vi "TIO Data Stream Parse timebase Info.vi"(8 "timebases in":T2(array[cluster]), 11 "timebase info raw":string="\u0001\u0000\u0001\u0002 \u0006\u001c\u0006\u0000\u0000\u0000\u0000Ð\u0012\u0013\u0000è\u0003\u0000\u0000\u0001\u0000\u0000\u0000\u0017·Q8\u0001\u0000\u0000\u0000?\u0000\u0016\u0000\u0011P6W462 ") -> (0 "timebases out":T2(array[cluster]))   [LabVIEW 2012]
panel:
  out "timebase info":T1
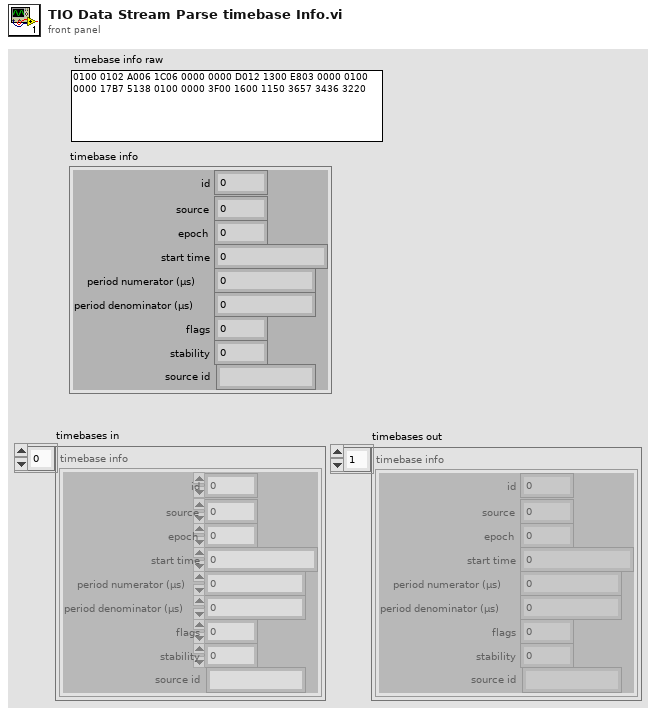
[diagram p1: front panel]
types:
  T1 = cluster{"id":u16, "source":u8, "epoch":u8, "start time":u64, "period numerator (µs)":u32, "period denominator (µs)":u32, "flags":u32, "stability":sgl, "source id":string}
  T2 = cluster{"id":u16, "source":u8, "epoch":u8, "start time":u64, "period numerator (µs)":u32, "period denominator (µs)":u32, "flags":u32, "stability":sgl, "source id":string}[]
  T3 = enum16{"big-endian, network order", "native, host order", "little-endian"}
  T4 = cluster{"u16":u16, "u8":u8, "u8":u8, "u64":u64, "u32":u32, "u32":u32, "u32":u32, "f32":sgl}
  T5 = cluster{"u16":u16, "u8":u8, "u8":u8, "u64":u64, "u32":u32, "u32":u32, "u32":u32, "f32":sgl, string}
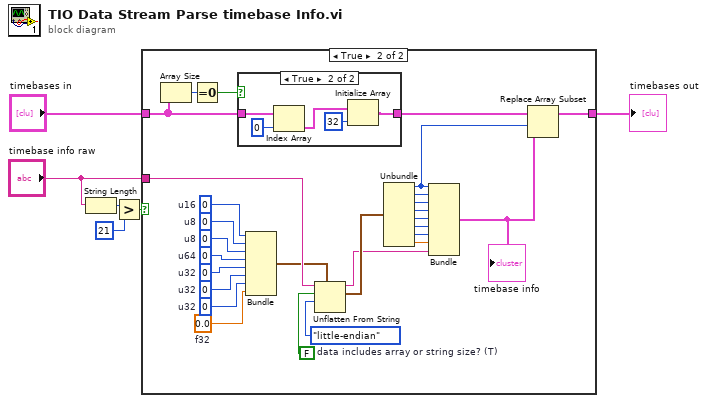
[diagram p0: block diagram]
diagram:
  n1 = String Length(string="timebase info raw") -> (length=w5:i32)
  n2 = Greater?(x=w5, y=21) -> (0:w4:bool)
  n3 = case shown="True" w4 {
    tunnel: "timebase info raw" -> [_ w35]
    tunnel: "timebases in" -> [w7 w12]
    tunnel: [w7 w10] -> w1
    frame False {
    }
    frame True {
      w27 = sgl 0.0  # f32
      w25 = u32 0  # u32
      w28 = u32 0  # u32
      w29 = u32 0  # u32
      w30 = u64 0  # u64
      w31 = u8 0  # u8
      w32 = u8 0  # u8
      w24 = u16 0  # u16
      w34 = FALSE  # data includes array or string size? (T)
      n4 = Array Size(array=w12) -> (size(s)=w14:i32)
      n5 = Equal To 0?(x=w14) -> (x = 0?=w13:bool)
      n6 = case shown="True" w13 {
        tunnel: [w36 w41] -> w11
        tunnel: w12 -> [w36 w39]
        frame False {
        }
        frame True {
          n7 = Index Array(array=w39, index=0) -> (element=w37:T1)
          n8 = Initialize Array(w37, 32 ("dimension size")) -> (w41:T2)
        }
      }
      n9 = Bundle("u16"=w24, "u8"=w32, "u8"=w31, "u64"=w30, "u32"=w29, "u32"=w28, "u32"=w25, "f32"=w27) -> (w26:T4)  [unwired: 1 in]
      n10 = Unflatten From String(type=w26, binary string=w35, data includes array or string size? (T)=w34, byte order (0:big-endian, network order)=T3."little-endian") -> (rest of the binary string=w15:string, value=w23:T4)  [unwired: 1 in, 1 out]
      n11 = Unbundle(w23) -> ("u16"=w9:u16, "u8"=w22:u8, "u8"=w21:u8, "u64"=w20:u64, "u32"=w19:u32, "u32"=w18:u32, "u32"=w17:u32, "f32"=w16:sgl)
      n12 = Bundle("u16"=w9, "u8"=w22, "u8"=w21, "u64"=w20, "u32"=w19, "u32"=w18, "u32"=w17, "f32"=w16, w15) -> (w8:T5)  [unwired: 1 in]
      "timebase info" <- w8
      n13 = Replace Array Subset(array=w11, new element=w8, index=w9) -> (w10:T2)
    }
  }
  "timebases out" <- w1
